vi "SPM100 control no loop v3.3.vi"(0 "VISA resource in":refnum<visa-resource-name>, 1 "Time to run (sec.)":dbl=26.086956521739133 format="%.1f", 2 "Max volume":dbl=0.0625, 5 "Pump No.":i8=3, 7 "Syringe size":dbl=4.7, 9 "Infuse/\nWithdraw":bool=TRUE caption="Push/Pull", 11 "error in":errorcluster, 12 "Flow rate":dbl=1.0, 13 "FlowRateUnit":u32(ring) items=["ml/min", "ml/hr", "ul/min", "ul/hr"]) -> (4 "VISA resource name out":refnum<visa-resource-name>, 6 "Closing":bool, 8 "dV":dbl, 15 "error out":errorcluster)   [LabVIEW 2014]
doc: "Non-initialised version of the SPM 100 pump controller.\nThis unlooped sub-vi allows control of the pump for sequential environment change without having to resort to the Camtech provided proprietary software. \nAll control inputs needs to be provided, including an initialised Visa reference, before invoking this routine."
uses:
  <vilib>/Platform/TimedLoop/XDataNode/timing_clust.ctl
  <vilib>/Platform/TimedLoop/XDataNode/nitl_modes.ctl
  <vilib>/Platform/TimedLoop/XDataNode/wakeup.ctl
  <vilib>/platform/TimedLoop/XDataNode/XDataNode.xnode
  <vilib>/Platform/TimedLoop/XDataNode/XDNodeRunTimeDep.lvlib
panel:
  out "Time run":dbl
  out "F":dbl
  in  "Reset":bool
  out "return count":u32
  in  "Close":bool
  out "Stop pressed":bool
  out "Remaining time (sec.)":dbl=2.0 format="%.1f"
  in  "Stop":bool
  out "Remaining volume":dbl(slide)=100.0 scale=0.0..100.0 scale format="%.0f%%"
  out "VolumeUnit":string="ml"
  in  "Run":bool
  # "SPM 100 Syringe Pump - Automatic control"
  # "Status"
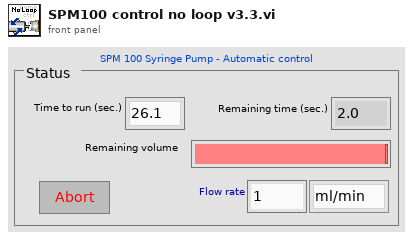
[diagram p1: front panel]
types:
  T1 = typedef "XDNodeRunTimeDep.lvlib/timing_clust.ctl" = cluster{"Expected End [f-1]":u64, "Actual End [f-1]":u64, "Finished Late? [f-1]":bool, "Expected End [i-1]":u64, "Actual End [i-1]":u64, "Finished Late? [i-1]":bool, "Expected Start [i]":u64, "Actual Start [i]":u64, "Expected Start [f]":u64, "Actual Start [f]":u64, "Source Name":string, "Structure Name":string, "Period":i64, "Deadline":i64, "Offset":i64, "Start":i64, "Priority":i32, "Timeout":i32, "Mode":T2, "Wakeup Reason":T3, "Error":errorcluster, "Source Type":string, "Secondary Source Type":string, "Global End Time":u64, "Global Start Time":u64, "Frame Duration":u64, "Iteration Duration":u64, "Assigned CPU":i32, "I/O Scan Engine Mode":u32}
  T2 = typedef "XDNodeRunTimeDep.lvlib/nitl_modes.ctl" = enum32{"No Change", "Process missed periods, maintain original phase", "Discard missed periods, maintain original phase", "Process missed periods, ignore original phase", "Discard missed periods, ignore original phase"}
  T3 = typedef "XDNodeRunTimeDep.lvlib/wakeup.ctl" = enum32{"Normal", "Aborted", "Asynchronous wakeup", "Timing source error", "Timed loop error", "Timeout"}
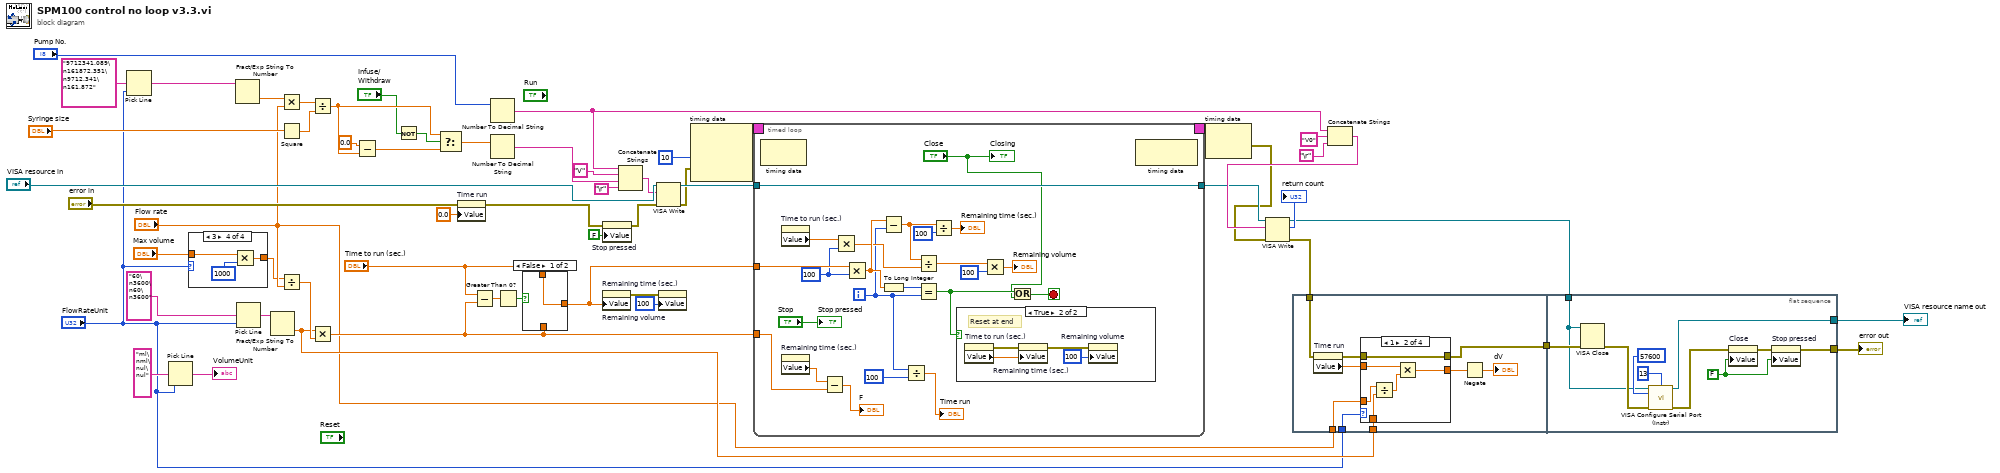
[diagram p0: block diagram]
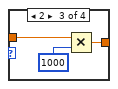
[diagram p4: hidden frame]
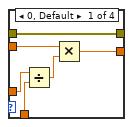
[diagram p5: hidden frame]
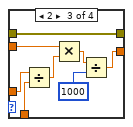
[diagram p6: hidden frame]
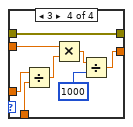
[diagram p7: hidden frame]
diagram:
  n1 = Pick Line(multi-line string="9712341.089\n161872.351\n9712.341\n161.872", line index="FlowRateUnit") -> (output string=w43:string)  [unwired: 1 in]
  n2 = Pick Line(multi-line string="ml\nml\nul\nul", line index="FlowRateUnit") -> (output string=→"VolumeUnit":string)  [unwired: 1 in]
  n3 = case shown="3" "FlowRateUnit" {
    tunnel: [w58 w59 w62 w65] -> w2
    tunnel: "Max volume" -> [w58 w59 w60 w63]
    frame 0, Default {
    }
    frame 1 {
    }
    frame 2 {
      n4 = Multiply(x=w60, y=1000) -> (x*y=w62:dbl)
    }
    frame 3 {
      n5 = Multiply(x=w63, y=1000) -> (x*y=w65:dbl)
    }
  }
  n6 = Fract/Exp String To Number(string=w43) -> (number=w42:dbl)  [unwired: 3 in, 1 out]
  n7 = Pick Line(multi-line string="60\n3600\n60\n3600", line index="FlowRateUnit") -> (output string=w40:string)  [unwired: 1 in]
  n8 = Fract/Exp String To Number(string=w40) -> (number=w9:dbl)  [unwired: 3 in, 1 out]
  n9 = Multiply(x=w42, y="Flow rate") -> (x*y=w53:dbl)
  n10 = Square(x="Syringe size") -> (x^2=w52:dbl)
  n11 = Divide(x=w2, y="Flow rate") -> (x/y=w47:dbl)
  n12 = Divide(x=w53, y=w52) -> (x/y=w49:dbl)
  n13 = Multiply(x=w9, y=w47) -> (x*y=w18:dbl)
  n14 = Subtract(x=0.0, y=w49) -> (x-y=w50:dbl)
  n15 = Not(x="Infuse/\nWithdraw") -> (.not. x?=w37:bool)
  n16 = Select(t=w49, s=w37, f=w50) -> (s? t:f=w51:dbl)
  n17 = property on="Time run" class="DigNum (strict)"(error in="error in", "Value"=0.0 ("Time run")) -> (error out=w12:errorcluster)  [unwired: 1 in, 1 out]
  n18 = Subtract(x="Time to run (sec.)", y=w18) -> (x-y=w20:dbl)
  n19 = Number To Decimal String(number="Pump No.") -> (decimal integer string=w57:string)  [unwired: 1 in]
  n20 = Number To Decimal String(number=w51) -> (decimal integer string=w39:string)  [unwired: 1 in]
  n21 = Greater Than 0?(x=w20) -> (x > 0?=w19:bool)
  n22 = case shown="False" w19 {
    tunnel: w18 -> [_ w67]
    tunnel: "Time to run (sec.)" -> [w66 _]
    tunnel: [w66 w67] -> w14
    frame False {
    }
    frame True {
    }
  }
  n23 = property on="Remaining time (sec.)" class="DigNum (strict)"("Value"=w14) -> (error out=w17:errorcluster)  [unwired: 2 in, 1 out]
  n24 = property on="Stop pressed" class="Bool (strict)"(error in=w12, "Value"=FALSE ("Stop")) -> (error out=w22:errorcluster)  [unwired: 1 in, 1 out]
  n25 = Concatenate Strings(w57, "V" ("string"), w39, "\r") -> (w33:string)
  n26 = VISA Write(VISA resource name="VISA resource in", write buffer=w33, error in (no error)=w22) -> (VISA resource name out=w34:refnum<visa-resource-name>, error out=w24:errorcluster)  [unwired: 1 out]
  n27 = property on="Remaining volume" class="Slide (strict)"(error in=w17, "Value"=100 ("Volume Remain  (%)")) -> ()  [unwired: 1 in, 2 out]
  n28 = node-c288 ("Input Node")(u32 10 ("millisecond multiple"), w24) -> (w36:T1)  [unwired: 1 in]
  n29 = timed-loop {
    tunnel: [w90] -> w27
    tunnel: w34 -> [w90]
    tunnel: w14 -> [w85]
    timing: w36 -> [_]
    timing-out: [_] -> w35
    tunnel: w18 -> [w73]
    i -> [w69]
    stop <- w80 stop-if-true
    w77 = 100
    n30 = node-c288() -> ()  [unwired: 1 in, 1 out]
    n31 = property on="Time to run (sec.)" class="DigNum (strict)"() -> ("Value"=w78:dbl)  [unwired: 2 in, 2 out]
    n32 = property on="Remaining time (sec.)" class="DigNum (strict)"() -> ("Value"=w72:dbl)  [unwired: 2 in, 2 out]
    n33 = Subtract(x=w72, y=w73) -> (x-y=→"F":dbl)
    n34 = Multiply(x=w78, y=w77) -> (x*y=w76:dbl)
    n35 = Multiply(x=w85, y=w77) -> (x*y=w84:dbl)
    n36 = Subtract(x=w84, y=w69) -> (x-y=w88:dbl)
    n37 = To Long Integer(number=w84) -> (32bit integer=w86:i32)
    n38 = Divide(x=w69, y=100) -> (x/y=→"Time run":dbl)
    n39 = Divide(x=w88, y=w76) -> (x/y=w81:dbl)
    n40 = Equal?(x=w86, y=w69) -> (x = y?=w79:bool)
    n41 = Divide(x=w88, y=100) -> (x/y=→"Remaining time (sec.)":dbl)
    n42 = case shown="True" w79 {
      frame False {
      }
      frame True {
        # "Reset at end"
        n43 = property on="Time to run (sec.)" class="DigNum (strict)"() -> (error out=w94:errorcluster, "Value"=w93:dbl)  [unwired: 2 in, 1 out]
        n44 = property on="Remaining time (sec.)" class="DigNum (strict)"(error in=w94, "Value"=w93) -> (error out=w92:errorcluster)  [unwired: 1 in, 1 out]
        n45 = property on="Remaining volume" class="Slide (strict)"(error in=w92, "Value"=100 ("Volume Remain  (%)")) -> ()  [unwired: 1 in, 2 out]
      }
    }
    n46 = Multiply(x=w81, y=100) -> (x*y=→"Remaining volume":dbl)
    n47 = Or(x=w79, y="Close") -> (x .or. y?=w80:bool)
    n48 = node-c288() -> ()  [unwired: 1 in, 1 out]
    "Stop pressed" <- "Stop"
    "Closing" <- "Close"
  }
  n49 = node-c288(w35) -> (w21:errorcluster)
  n50 = flat-sequence {
    tunnel: w10 -> [w103]
    tunnel: "FlowRateUnit" -> [w101]
    tunnel: w9 -> [w100]
    tunnel: "Flow rate" -> [w99]
    tunnel: [w105] -> w7
    tunnel: [w134] -> w4
    tunnel: w7 -> [w137]
    tunnel: w6 -> [w136]
    tunnel: [w135] -> w5
    frame #0 {
      n51 = property on="Time run" class="DigNum (strict)"(error in=w103) -> (error out=w102:errorcluster, "Value"=w104:dbl)  [unwired: 1 in, 1 out]
      n52 = case shown="1" w101 {
        tunnel: w100 -> [w108 w117 w125 w133]
        tunnel: w99 -> [w109 w116 w124 w132]
        tunnel: w104 -> [w110 w115 w123 w131]
        tunnel: [w107 w113 w122 w130] -> w98
        tunnel: w102 -> [w106 w112 w118 w126]
        tunnel: [w106 w112 w118 w126] -> w105
        frame 0, Default {
          n53 = Divide(x=w109, y=w108) -> (x/y=w111:dbl)
          n54 = Multiply(x=w110, y=w111) -> (x*y=w107:dbl)
        }
        frame 1 {
          n55 = Divide(x=w116, y=w117) -> (x/y=w114:dbl)
          n56 = Multiply(x=w115, y=w114) -> (x*y=w113:dbl)
        }
        frame 2 {
          n57 = Divide(x=w124, y=w125) -> (x/y=w120:dbl)
          n58 = Multiply(x=w123, y=w120) -> (x*y=w121:dbl)
          n59 = Divide(x=w121, y=1000) -> (x/y=w122:dbl)
        }
        frame 3 {
          n60 = Divide(x=w132, y=w133) -> (x/y=w128:dbl)
          n61 = Multiply(x=w131, y=w128) -> (x*y=w129:dbl)
          n62 = Divide(x=w129, y=1000) -> (x/y=w130:dbl)
        }
      }
      n63 = Negate(x=w98) -> (-x=→"dV":dbl)
    }
    frame #1 {
      w139 = FALSE ("Quit")
      n64 = VISA Close(VISA resource name=w136, error in (no error)=w137) -> (error out=w142:errorcluster)
      n65 = call <vilib>:"VISA Configure Serial Port (Instr).vi"("VISA resource name"=w136, "termination char\n(0xA = '\\n' = LF)"=u8 13 ("termination char\n(0xD = '\\r' = CR)"), "baud rate (9600)"=u32 57600 ("baud rate"), "error in (no error)"=w142) -> ("VISA resource name out"=w135:refnum<visa-resource-name>, "error out"=w143:errorcluster)  [unwired: 10 in]
      n66 = property on="Close" class="Bool (strict)"(error in=w143, "Value"=w139) -> (error out=w138:errorcluster)  [unwired: 1 in, 1 out]
      n67 = property on="Stop pressed" class="Bool (strict)"(error in=w138, "Value"=w139) -> (error out=w134:errorcluster)  [unwired: 1 in, 1 out]
    }
  }
  n68 = Concatenate Strings(w57, "V0" ("Write Command 2"), "\r") -> (w28:string)
  n69 = VISA Write(VISA resource name=w27, write buffer=w28, error in (no error)=w21) -> (VISA resource name out=w6:refnum<visa-resource-name>, return count=→"return count":u32, error out=w10:errorcluster)
  "VISA resource name out" <- w5
  "error out" <- w4
